vi "Add gRPC Server to Map.vi"(8 "error in (no error)":errorcluster, 10 "gRPC Server Class":refnum<class "ServiceBase.lvclass">, 11 "CIFLauncher in":refnum<class "CIFLauncher.lvclass">) -> (0 "error out":errorcluster, 3 "CIFLauncher out":refnum<class "CIFLauncher.lvclass">)   [LabVIEW 2021, in "CIFLauncher.lvclass"]
uses:
  CIFLauncher.lvclass
  CIFLauncher.lvclass/CIFLauncher.ctl
  <vilib>/gRPC/LabVIEW gRPC Servicer/ServiceBase/ServiceBase.lvclass
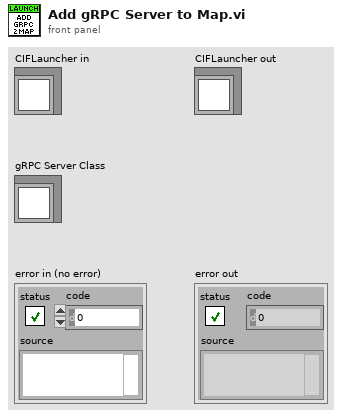
[diagram p1: front panel]
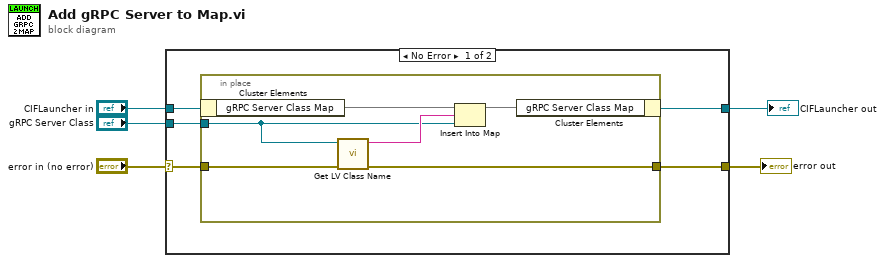
[diagram p0: block diagram]
diagram:
  n1 = case shown="No Error" "error in (no error)" {
    selector: "error in (no error)" -> [w8 w18]
    tunnel: [w7 w18] -> w3
    tunnel: [w9 w17] -> w2
    tunnel: "CIFLauncher in" -> [w10 w17]
    tunnel: "gRPC Server Class" -> [w6 _]
    frame No Error {
      n2 = in-place {
        in-place-border: w8 -> [w14]
        in-place-border: [w13] -> w7
        in-place-border: w6 -> [w11]
        n3 = in-place-cluster #1(w10) -> ("gRPC Server Class Map"=w16:map{string, refnum<class "ServiceBase.lvclass">})
        n4 = call <vilib>:"Get LV Class Name.vi"("error in (no error)"=w14, "object"=w11) -> ("error out"=w13:errorcluster, "class name"=w12:string)  [unwired: 8 in]
        n5 = Insert Into Map(map in=w16, key=w12, value=w11) -> (map out=w15:map{string, refnum<class "ServiceBase.lvclass">})  [unwired: 2 out]
        n6 = in-place-cluster #1("gRPC Server Class Map"=w15) -> (w9:refnum<class "CIFLauncher.lvclass">)
      }
    }
    frame Error {
    }
  }
  "error out" <- w3
  "CIFLauncher out" <- w2
